vi "1-x.vi"(5 "x":sgl) -> (6 "1-x":sgl)   [LabVIEW 2016]
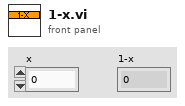
[diagram p1: front panel]
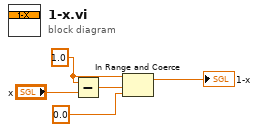
[diagram p0: block diagram]
diagram:
  w3 = sgl 1.0 ("x")
  n1 = Subtract(x=w3, y="x") -> (x-y=w4:sgl)
  n2 = In Range and Coerce(upper limit=w3, x=w4, lower limit=sgl 0.0) -> (coerced(x)=→"1-x":sgl)  [unwired: 1 out]
